vi "ValveControl-externalConnection.vi"() -> ()   [LabVIEW 2016]
uses:
  Classes/Controllers/I-O/Copy of NI-DAQ Folder/NI-DAQ.lvclass
panel:
  in  "values":bool[](array[boolean])=[TRUE]
  in  "indices":i32[](array[numeric])=[0]
  in  "DAQ Module":i32
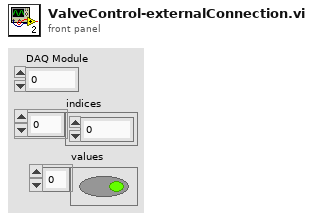
[diagram p1: front panel]
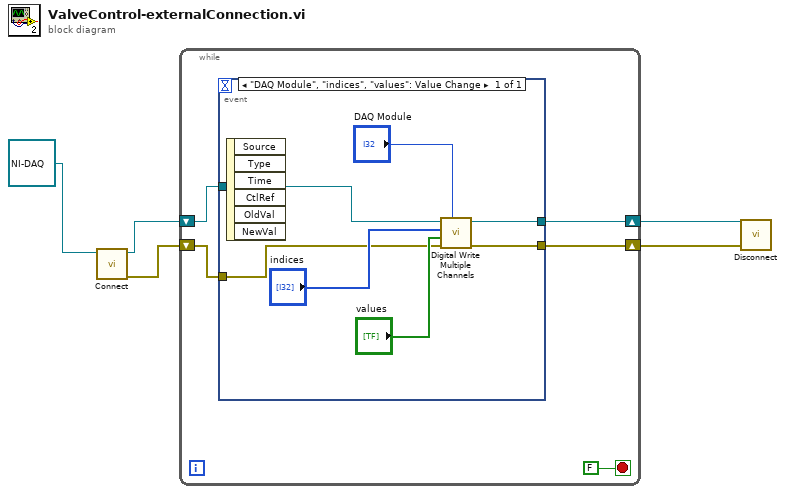
[diagram p0: block diagram]
diagram:
  n1 = call-dynamic "Connect.vi"("NI-DAQ in"=refnum<class "NI-DAQ.lvclass"> refnum ("NI-DAQ.lvclass")) -> ("error out"=w4:errorcluster, "NI-DAQ out"=w5:refnum<class "NI-DAQ.lvclass">)  [unwired: 9 in]
  n2 = while {
    shift-right: [w8] -> w2
    shift-left: w5 -> [w10]
    shift-right: [w7] -> w1
    shift-left: w4 -> [w9]
    stop <- FALSE stop-if-true
    n3 = event shown="[0] \"DAQ Module\", \"indices\", \"values\": Value Change" {
      selector: _ -> [_]
      dyn-events: _ -> [_]
      timeout: _ -> [_]
      tunnel: w10 -> [w14]
      tunnel: w9 -> [w13]
      tunnel: [w12] -> w8
      tunnel: [w11] -> w7
      event "DAQ Module", "indices", "values": Value Change {
        n4 = event-data() -> ()  [unwired: 1 in, 6 out]
        n5 = call-dynamic "Digital Write Multiple Channels.vi"("DAQ Module"="DAQ Module", "error in (no error)"=w13, "Values"="values", "Indices"="indices", "NI-DAQ in"=w14) -> ("error out"=w11:errorcluster, "NI-DAQ out"=w12:refnum<class "NI-DAQ.lvclass">)  [unwired: 5 in]
      }
    }
  }
  n6 = call-dynamic "Disconnect.vi"("error in (no error)"=w1, "I-O in"=w2) -> ()  [unwired: 8 in, 1 out]
